vi "rs3 get profiles count.vi"(8 "error in":errorcluster, 11 "Profiles_list":u64) -> (0 "error out":errorcluster, 1 "Profiles_list_out":u64, 2 "Profiles count":i32, 3 "error":u64)   [LabVIEW 2018, in "libRealSense3.lvlib"]
doc: "Returns the number of PROFILES that exist in the PROFILE LIST of the SENSOR"
uses:
  libRealSense3.lvlib
  realsense2.dll
panel:
  # "RS3 Get Stream Profiles Count"
  # "(C) Intel Corp. 2017,  AGJ"
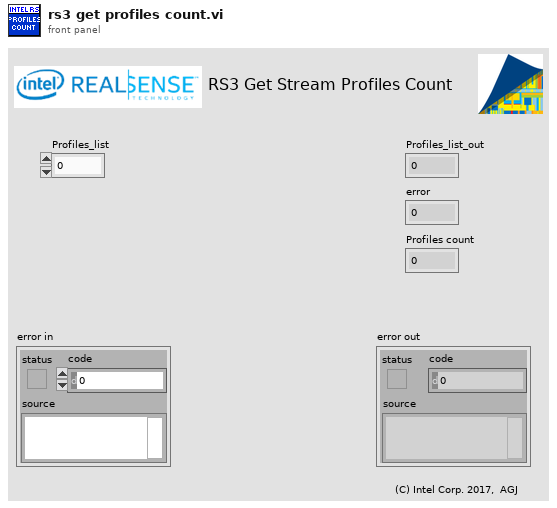
[diagram p1: front panel]
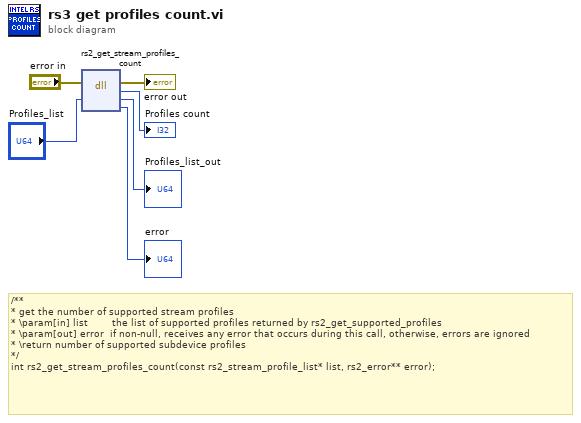
[diagram p0: block diagram]
diagram:
  # "/**\n* get the number of supported stream profiles\n* \\param[in] list        the list of supported profiles returned by rs2_get_supported_profiles\n* \\param[out] error  if non-null, receives any error that occurs during this call, otherwise, errors are ignored\n* \\return number of supported subdevice profiles\n*/\nint rs2_get_stream_profiles_count(const rs2_stream_profile_list* list, rs2_error** error);"
  n1 = dll-call lib="C:/Users/aaron.jencks/Documents/Temp/realsense_labview_sdk/RealSense SDK2.11.0 for LabVIEW/realsense2.dll" fn="rs2_get_stream_profiles_count"(error in="error in", "Profiles list"="Profiles_list") -> (error out=→"error out":errorcluster, "Stream profiles count"=→"Profiles count":i32, "Profiles list"=→"Profiles_list_out":u64, "error"=→"error":u64)  [unwired: 3 in, 1 out]
